vi "Alarms.vi"() -> ()   [LabVIEW 2013]
panel:
  in  "TI-342 HIHI":dbl=375.0
  out "String 2":string
  out "String":string
  in  "TI_502 HIHI":dbl
  in  "TI_502 HI":dbl=inf
  in  "TI_151 HIHI":dbl
  in  "TI_151 HI":dbl
  out "String 3":string
  in  "TI_501 HIHI":dbl
  in  "TI_501 HI":dbl
  in  "TI_503 HIHI":dbl
  in  "TI_503 HI":dbl
  out "String 4":string
  in  "PI_501 HIHI":dbl
  in  "PI_501 HI":dbl
  out "String 5":string
  in  "PI_600 HIHI":dbl
  in  "PI_600 HI":dbl
  in  "PI_621 HIHI":dbl
  in  "PI_621 HI":dbl
  out "String 6":string
  out "String 7":string
  in  "PI_641 HIHI":dbl
  in  "PI_641 HI":dbl
  in  "TI_510 HIHI":dbl
  in  "TI_510 HI":dbl
  in  "TI_510 LO":dbl
  in  "TI_510 LOLO":dbl
  in  "TI_520 HIHI":dbl
  in  "TI_520 HI":dbl
  in  "TI_520 LO":dbl
  in  "TI_520 LOLO":dbl
  out "String 8":string
  out "String 9":string
  out "String 10":string
  in  "TI_530 HIHI":dbl
  in  "TI_530 HI":dbl
  in  "TI_530 LO":dbl
  in  "TI_530 LOLO":dbl
  out "String 11":string
  in  "TI_601 HIHI":dbl
  in  "TI_601 HI":dbl
  out "String 12":string
  in  "TI_602 HIHI":dbl
  in  "TI_610 HIHI":dbl
  in  "TI_602 HI":dbl
  in  "TI_610 HI":dbl
  out "String 13":string
  out "String 14":string
  in  "TI_620 HIHI":dbl
  in  "TI_620 HI":dbl
  out "String 15":string
  in  "FC_101 HIHI":dbl
  in  "FC_101 HI":dbl
  in  "FC_101 LO":dbl
  in  "FC_101 LOLO":dbl
  out "String 16":string
  in  "TI_341 LOLO":dbl
  in  "TI_341 LO":dbl
  out "String 17":string
  in  "PI_341 HI":dbl
  in  "PI_341 HIHI":dbl
  out "String 18":string
  in  "PI_131 LOLO":dbl
  in  "PI_131 LO":dbl
  out "String 19":string
  in  "Feed Hopper Lo":dbl
  out "String 20":string
  in  "PI_201 HIHI":dbl
  in  "PI_201 HI":dbl
  out "String 22":string
  in  "PI_201 LOLO":dbl
  in  "V200 O2 HIHI":dbl
  in  "PI_201 LO":dbl
  in  "V200 O2 HI":dbl
  out "String 23":string
  in  "V200 LEL HIHI":dbl
  in  "V200 LEL HI":dbl
  in  "MFC_111 LO":dbl
  in  "MFC_111 HI":dbl
  out "String 24":string
  out "String 25":string
  in  "MFC_121 Hi":dbl
  in  "MFC_121 LO":dbl
  out "String 26":string
  in  "TI_201 HIHI":dbl
  in  "PI_701 LO":dbl
  in  "PI_411 LO":dbl
  in  "TI_201 HI":dbl
  in  "V600 O2 HIHI":dbl
  in  "V600 O2 HI":dbl
  out "String 28":string
  out "String 29":string
  out "String 30":string
  out "String 27":string
  out "String 31":string
  in  "PI_701 LOLO":dbl
  in  "PI_701 HIHI":dbl
  in  "PI-701 HI":dbl
  in  "PI_421 LO":dbl
  in  "PI_411 HI":dbl
  in  "PI_421 HI":dbl
  in  "Save to file":bool
  in  "PI-151 HIHI":dbl
  in  "PI-151 HI":dbl
  in  "Load":bool=TRUE
  out "String 32":string
  out "String 33":string
  out "String 21":string
  in  "TI-741 HIHI":dbl
  in  "TI_741 HI":dbl
  out "String 34":string
  in  "TI-742 HI":dbl
  in  "TI-742 HIHI":dbl
  out "String 35":string
  in  "TI-743 HI":dbl
  in  "TI-743 HIHI":dbl
  out "String 36":string
  in  "TI-744 HI":dbl
  in  "TI-744 HIHI":dbl
  out "String 37":string
  in  "TI-745 HIHI":dbl
  in  "TI-745 HI":dbl
  in  "TI-746 HIHI":dbl
  out "String 38":string
  in  "TI-746 HI":dbl
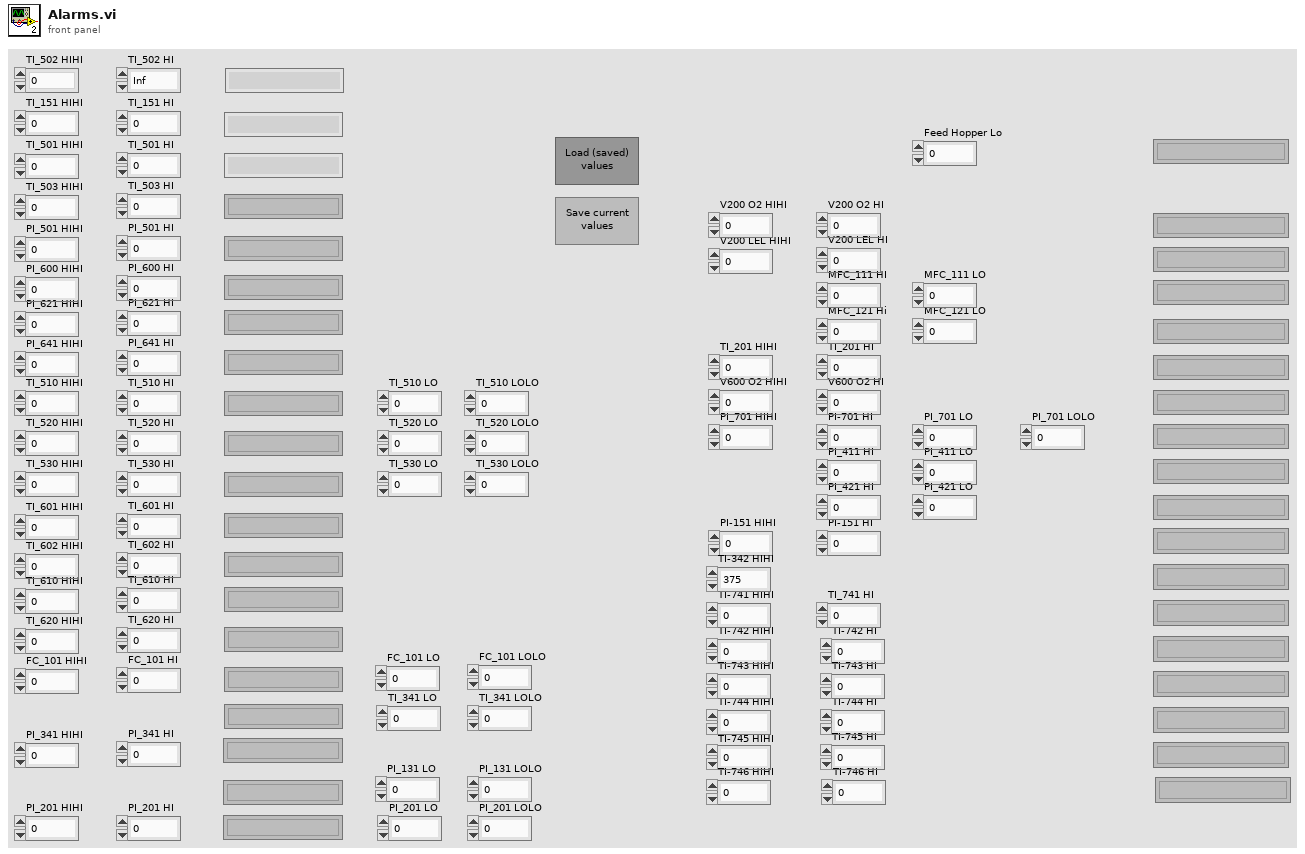
[diagram p1: front panel]
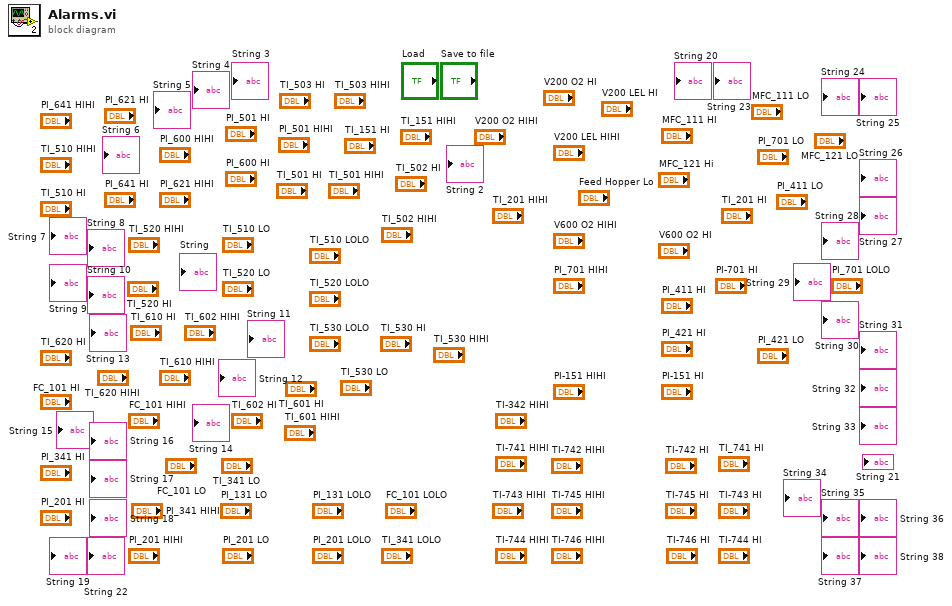
[diagram p0: block diagram]
diagram:
